vi "Pos_Find Global Position of Control.vi"(8 "Error":errorcluster, 9 "Control Name":string, 11 "VI":refnum<vi>) -> (0 "Error Out":errorcluster, 2 "Found Out":bool, 3 "Global Position Out":T1)   [LabVIEW 2024]
uses:
  <vilib>/Utility/miscctls.llb/LVRectTypeDef.ctl
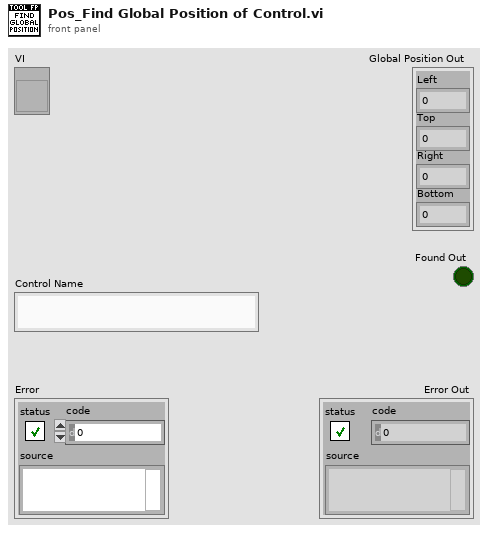
[diagram p1: front panel]
types:
  T1 = typedef "LVRectTypeDef.ctl" = cluster{"Left":i16, "Top":i16, "Right":i16, "Bottom":i16}
  T2 = typedef "LVPositionTypeDef.ctl" = cluster{"Left":i32, "Top":i32}
  T3 = typedef "LVBoundsTypeDef.ctl" = cluster{"Width":u32, "Height":u32}
  T4 = typedef "LVPointTypeDef.ctl" = cluster{"Horizontal":i16, "Vertical":i16}
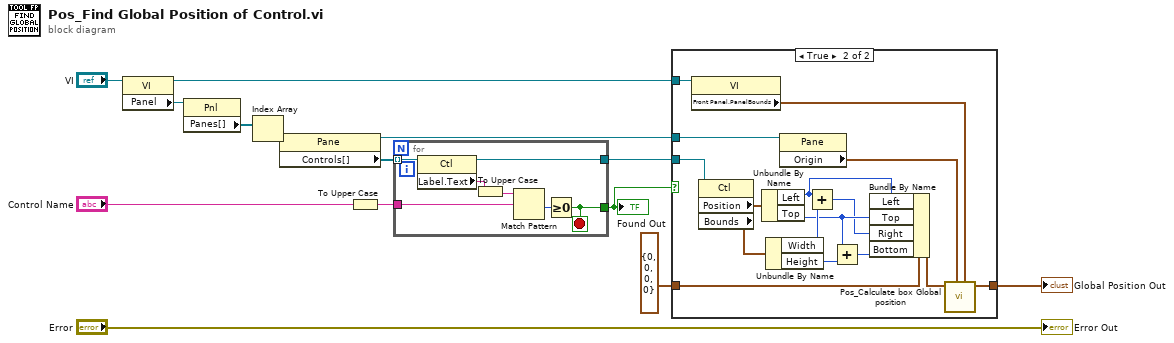
[diagram p0: block diagram]
diagram:
  n1 = property class="VI"(reference="VI") -> (reference out=w4:refnum<vi>, "Panel"=w12:refnum<vi>)  [unwired: 1 in, 1 out]
  n2 = property class="Pnl"(reference=w12) -> ("Panes[]"=w11:refnum<vi>[])  [unwired: 1 in, 2 out]
  n3 = Index Array(array=w11) -> (element=w9:refnum<vi>)  [unwired: 1 in]
  n4 = property class="Pane"(reference=w9) -> (reference out=w8:refnum<vi>, "Controls[]"=w7:refnum<vi>[])  [unwired: 1 in, 1 out]
  n5 = To Upper Case(1:"Control Name") -> (0:w5:string)
  n6 = for {
    tunnel: w7 -> [w21] mode=indexing
    tunnel: w5 -> [w19]
    tunnel: [w16] -> w1
    tunnel: [w15] -> w3
    stop <- w16 stop-if-true
    n7 = property class="Ctl"(reference=w21) -> (reference out=w15:refnum<vi>, "Label.Text"=w17:string)  [unwired: 1 in, 1 out]
    n8 = To Upper Case(1:w17) -> (0:w20:string)
    n9 = Match Pattern(string=w20, regular expression=w19) -> (offset past match=w18:i32)  [unwired: 1 in, 3 out]
    n10 = Greater Or Equal To 0?(x=w18) -> (x >= 0?=w16:bool)
  }
  "Found Out" <- w1
  n11 = case shown="True" w1 {
    tunnel: [w22 w38] -> w13
    tunnel: w8 -> [_ w36]
    tunnel: w4 -> [_ w35]
    tunnel: w3 -> [_ w34]
    tunnel: T1 {"Left"=0, "Top"=0, "Right"=0, "Bottom"=0} ("Window") -> [w22 w29]
    frame False {
    }
    frame True {
      n12 = property class="VI"(reference=w35) -> ("Front Panel.PanelBounds"=w24:T1)  [unwired: 1 in, 2 out]
      n13 = property class="Ctl"(reference=w34) -> ("Position"=w33:T2, "Bounds"=w32:T3)  [unwired: 1 in, 2 out]
      n14 = Unbundle By Name(w33) -> ("Left"=w25:i32, "Top"=w28:i32)
      n15 = Unbundle By Name(w32) -> ("Width"=w31:u32, "Height"=w30:u32)
      n16 = property class="Pane"(reference=w36) -> ("Origin"=w23:T4)  [unwired: 1 in, 2 out]
      n17 = Add(x=w25, y=w31) -> (x+y=w27:u32)
      n18 = Add(x=w28, y=w30) -> (x+y=w26:u32)
      n19 = Bundle By Name(cluster=w29, "Left"=w25, "Top"=w28, "Right"=w27, "Bottom"=w26) -> (w37:T1)
      n20 = call "Pos_Calculate box Global position.vi"("Front Panel.PanelBounds"=w24, "Origin"=w23, "Pane Position"=w37) -> ("Global Position Out"=w38:T1)  [unwired: 7 in, 1 out]
    }
  }
  "Global Position Out" <- w13
  "Error Out" <- "Error"
